vi "Get All Algorithms Info.vi"(6 "Backend engine":T1, 8 "error in":errorcluster) -> (0 "error out":errorcluster, 3 "All Algorithms Info":T2[](array[typedef]))   [LabVIEW 2013]
doc: "Get informations on all available Algorithms."
uses:
  TD Algorithm Information.ctl
  TD Backend Engine.ctl
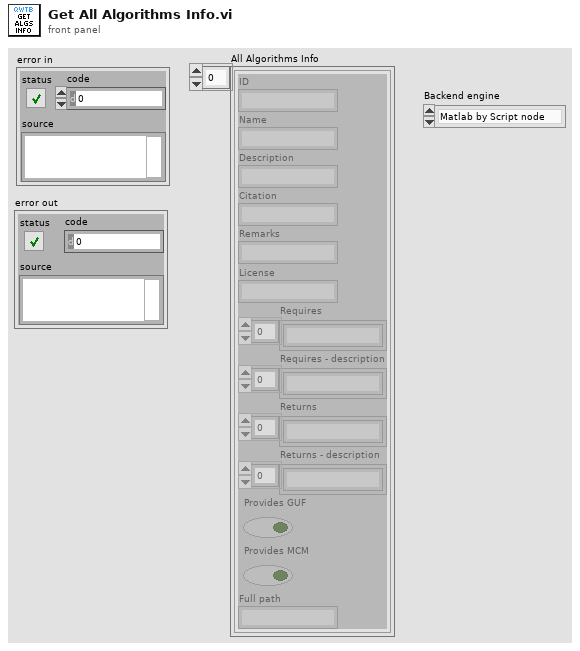
[diagram p1: front panel]
types:
  T1 = typedef "TD Backend Engine.ctl" = enum16{"Matlab by Script node", "GNU Octave by GOLPI"}
  T2 = typedef "TD Algorithm Information.ctl" = cluster{"ID":string, "Name":string, "Description":string, "Citation":string, "Remarks":string, "License":string, "Requires":string[], "Requires - description":string[], "Returns":string[], "Returns - description":string[], "Provides GUF":bool, "Provides MCM":bool, "Full path":string}
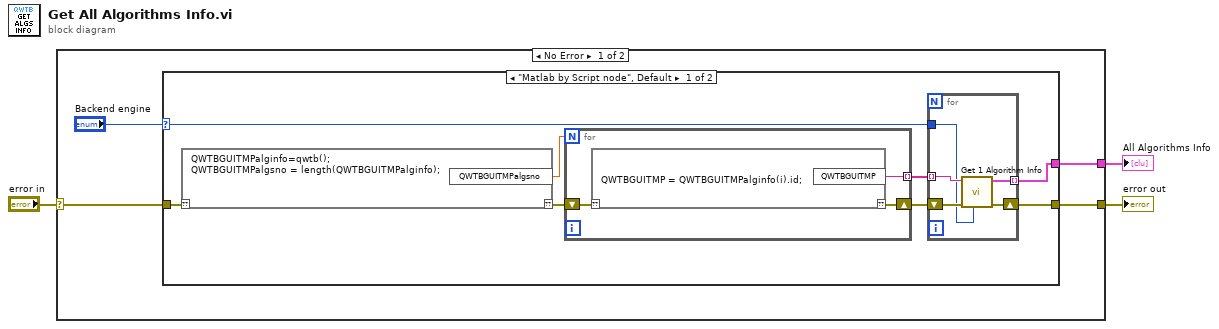
[diagram p0: block diagram]
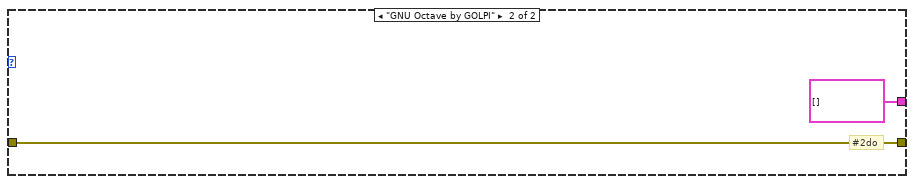
[diagram p2: hidden frame]
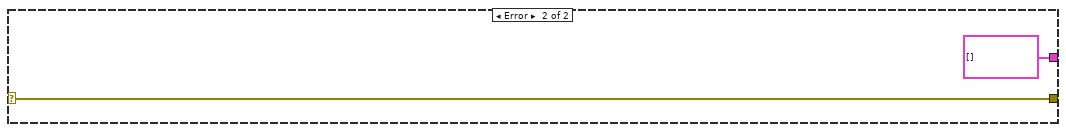
[diagram p3: hidden frame]
diagram:
  n1 = case shown="No Error" "error in" {
    selector: "error in" -> [w6 w27]
    tunnel: [w7 T2[] []] -> w3
    tunnel: [w5 w27] -> w1
    frame No Error {
      n2 = case shown="\"Matlab by Script node\", Default" "Backend engine" {
        selector: "Backend engine" -> [w8 _]
        tunnel: [w15 T2[] []] -> w7
        tunnel: w6 -> [w14 w25]
        tunnel: [w13 w25] -> w5
        frame "Matlab by Script node", Default {
          n3 = script code="QWTBGUITMPalginfo=qwtb();\nQWTBGUITMPalgsno = length(QWTBGUITMPalginfo);"("??"=w14) -> ("??"=w12:errorcluster, "QWTBGUITMPalgsno"=w9:dbl)
          n4 = for {
            N: w9 -> [_]
            tunnel: [w18] -> w10 mode=indexing
            shift-right: [w16] -> w11
            shift-left: w12 -> [w17]
            n5 = script code="QWTBGUITMP = QWTBGUITMPalginfo(i).id;"("??"=w17) -> ("??"=w16:errorcluster, "QWTBGUITMP"=w18:string)
          }
          n6 = for {
            tunnel: [w22] -> w15 mode=indexing
            shift-right: [w23] -> w13
            shift-left: w11 -> [w21]
            tunnel: w10 -> [w20] mode=indexing
            tunnel: w8 -> [w19]
            n7 = call "Get 1 Algorithm Info.vi"("Backend engine"=w19, "error in (no error)"=w21, "Algorithm ID"=w20) -> ("error out"=w23:errorcluster, "Algorithm Information"=w22:T2)  [unwired: 7 in]
          }
        }
        frame "GNU Octave by GOLPI" {
          # "#2do"
        }
      }
    }
    frame Error {
    }
  }
  "All Algorithms Info" <- w3
  "error out" <- w1
